vi "Unflatten From String.vi"(8 "error in (no error)":errorcluster, 10 "String":string, 11 "Serializer in":refnum<class "Serializer.lvclass">) -> (0 "error out":errorcluster, 2 "Record":refnum<class "Record.lvclass">, 3 "Serializer out":refnum<class "Serializer.lvclass">)   [LabVIEW 2017, in "Error Log.lvlib" / "Serializer.lvclass"]
uses:
  Serializer.lvclass
  Record/Record.lvclass
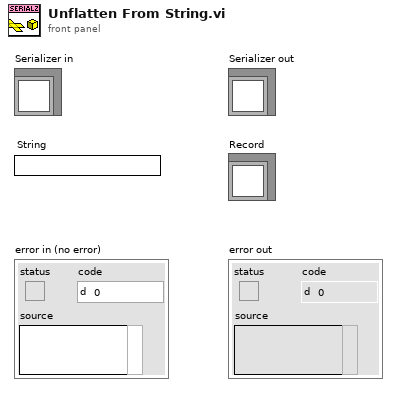
[diagram p1: front panel]
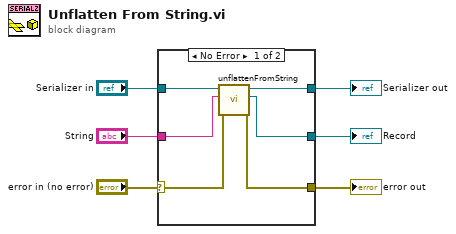
[diagram p0: block diagram]
diagram:
  n1 = case shown="No Error" "error in (no error)" {
    selector: "error in (no error)" -> [w10 w14]
    tunnel: [w9 w14] -> w5
    tunnel: [w11 w13] -> w3
    tunnel: "Serializer in" -> [w12 w13]
    tunnel: "String" -> [w8 _]
    tunnel: [w7 _] -> w1
    frame No Error {
      n2 = call-dynamic "unflattenFromString.vi"("error in (no error)"=w10, "String"=w8, "Serializer in"=w12) -> ("error out"=w9:errorcluster, "Record"=w7:refnum<class "Record.lvclass">, "Serializer out"=w11:refnum<class "Serializer.lvclass">)  [unwired: 6 in]
    }
    frame Error {
    }
  }
  "error out" <- w5
  "Serializer out" <- w3
  "Record" <- w1
